vi "5.4-6.7.3-What Server.vi"() -> ()   [LabVIEW 2010]
doc: "Creates a named service and listens on the first available port. Whenever a client connects to the service, it responds with a message containing joystick data. The VI can be stopped using the STOP button."
uses:
  6-OCU Neurons/6.0-Super Heart Beat.ctl
  5.7-UDP/5.7 LabVIEW Errors.ctl
  5.0-Global.vi
panel:
  out "Super Heart Beat":T1
  in  "error in":errorcluster={"status"=TRUE, "code"=0, "source"=""}
  out "error out":errorcluster
  in  "stop":bool
  out "Probably a hello string":string
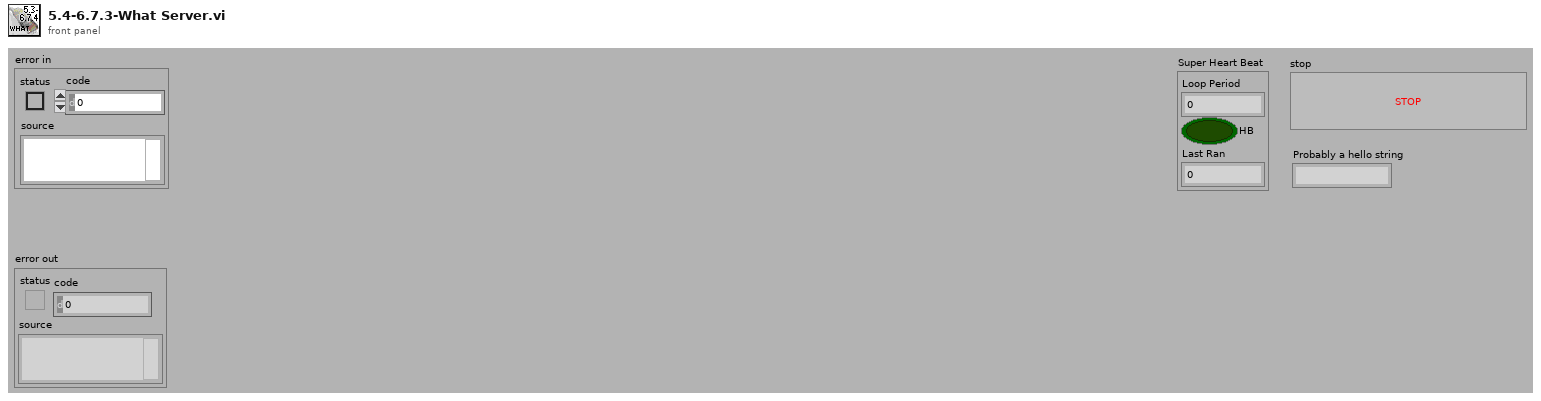
[diagram p1: front panel]
types:
  T1 = typedef "6.0-Super Heart Beat.ctl" = cluster{"Loop Period":u32, "HB":bool, "Last Ran":u32}
  T2 = typedef "6.3-What Reporting.ctl" = cluster{"LIDAR Data":T3}
  T3 = typedef "3.3.1-LIDAR Data Typedef.ctl" = cluster{"Angle array":dbl[], "Magnitude array ":dbl[]}
  T4 = typedef "5.7 LabVIEW Errors.ctl" = i32
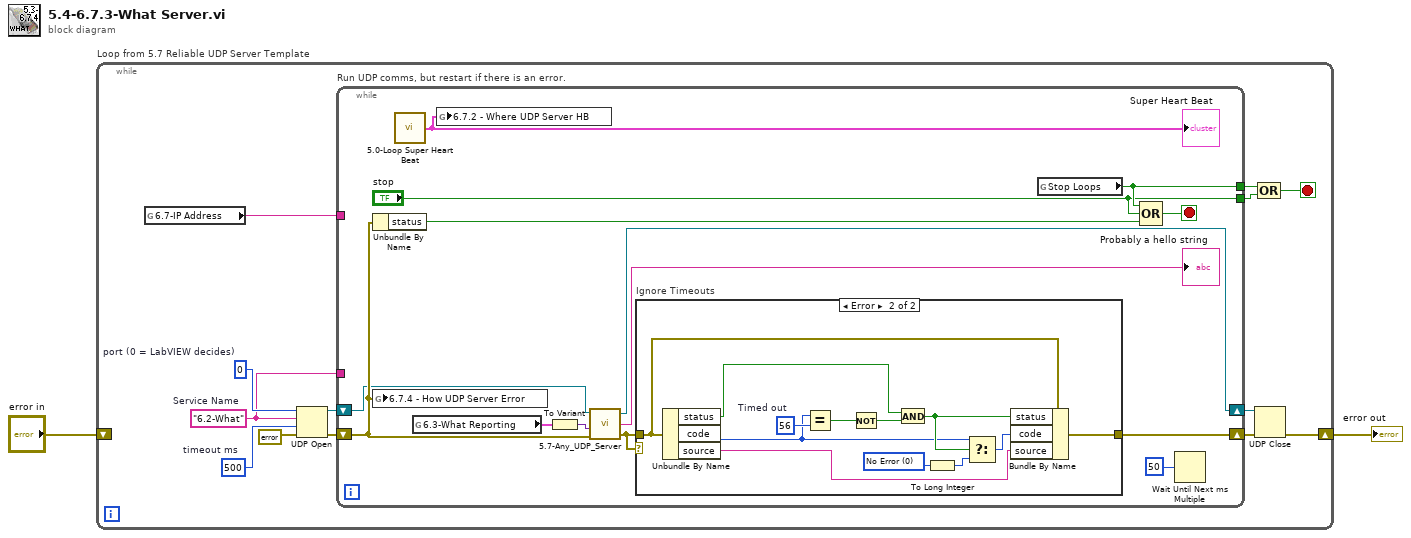
[diagram p0: block diagram]
diagram:
  n1 = while "Loop from 5.7 Reliable UDP Server Template" {
    shift-right: [w8] -> w1
    shift-left: "error in" -> [_]
    stop <- w13 stop-if-true
    w5 = 500  # timeout ms
    w7 = u16 0  # port (0 = LabVIEW decides)
    w6 = "6.2-What"  # Service Name
    n2 = global read "5.0-Global.vi" "6.7-IP Address"() -> (w4:string)
    n3 = UDP Open(8:errorcluster {"status"=FALSE, "code"=0, "source"=""} ("error in (no error)"), 9:w5, 10:w6, 11:w7) -> (port=w12:refnum<k16>, 0:w10:errorcluster)  [unwired: 1 in, 1 out]
    n4 = while "Run UDP comms, but restart if there is an error." {
      tunnel: w6 -> [_]
      tunnel: w4 -> [_]
      tunnel: [w27] -> w15
      tunnel: ["stop"] -> w14
      shift-right: [w20] -> w11
      shift-left: w12 -> [w21]
      shift-right: [w24] -> w9
      shift-left: w10 -> [w23]
      stop <- w29 stop-if-true
      n5 = Unbundle By Name(w23) -> ("status"=w25:bool)
      n6 = global write "5.0-Global.vi" "6.7.4 - How UDP Server Error"(w23) -> ()
      n7 = call "5.0-Loop Super Heart Beat.vi"() -> ("Super Heart Beat"=w16:T1)
      "Super Heart Beat" <- w16
      n8 = global read "5.0-Global.vi" "6.3-What Reporting"() -> (w17:T2)
      n9 = global write "5.0-Global.vi" "6.7.2 - Where UDP Server HB"(w16) -> ()
      n10 = To Variant(anything=w17) -> (Variant=w19:variant)
      n11 = call "5.7-Any_UDP_Server.vi"("error In"=w23, "Data in"=w19, "Connection ID"=w21) -> ("warning out"=w22:errorcluster, "data out"=→"Probably a hello string":string, "Connection ID out"=w20:refnum<k16>)  [unwired: 1 in]
      n12 = case "Ignore Timeouts" shown="Error" w22 {
        tunnel: w22 -> [w30 w42]
        tunnel: [w30 w41] -> w24
        frame No Error {
        }
        frame Error {
          w32 = T4 0 items=["No Error", "Argument Error", "Memory Full", "Out of Zone", "End of File", "File Already Open", "Generic File IO Error", "File Not Found", "File Permission Error", "Disk Full", "Duplicate Path", "Too Many Files Open", "Not Enabled", "Resource File Not Found", "Cannot Add Resource", "Resource Not Found", "Image Not Found", "Image Memory Error", "Pen Does Not Exist", "Config Bad Type", "Config Token Not Found", "Config Parse Error", "Config Memory Error", "Bad External Code Format", "Bad External Code Offset", "External Code Not Present", "Null Window", "Destroy Window Mixup", "Null Menu", "Print Aborted", "Bad Print Record", "Print Driver Error", "Windows Error During Print", "Memory Error During Print", "Print Dialog Error", "Generic Print Error", "Invalid Device Refnum", "Device Not Found", "Device Parameter Error", "Device Unit Error", "Can't Open Device", "Device Call Aborted", "Generic Error", "Cancelled By User", "Object ID Too Low", "Object ID Too High", "Object Not In Heap", "Unknown Heap", "Bad DefProc ID", "DefProc Not In Table", "Message Out Of Range", "Null Method", "Unknown Message", "Manager Call Not Supported", "Bad address", "Connection In progress", "Connection timed out", "Connection is already in progress", "Network attribute not supported", "Network error", "Address in use", "System out of memory", "Connection aborted", "Connection refused", "Connection is not connected", "Connection is already connected", "Connection closed", "Initialize error (interapplication manager)", "Bad occurrence", "Wait on unbound occurrence handler", "Occurrence queue overflow", "Bad path", "Semaphore not signaled", "Unrecognized type (interapplication manager)"] ("1st Error to Convert")
          w40 = 56  # Timed out
          n13 = Unbundle By Name(w42) -> ("status"=w37:bool, "code"=w35:i32, "source"=w33:string)
          n14 = Equal?(x=w35, y=w40) -> (x = y?=w39:bool)
          n15 = Not(x=w39) -> (.not. x?=w38:bool)
          n16 = And(x=w37, y=w38) -> (x .and. y?=w36:bool)
          n17 = To Long Integer(number=w32) -> (32bit integer=w31:T4)
          n18 = Select(t=w35, s=w36, f=w31) -> (s? t:f=w34:T4)
          n19 = Bundle By Name(cluster=w42, "status"=w36, "code"=w34, "source"=w33) -> (w41:errorcluster)
        }
      }
      n20 = global read "5.0-Global.vi" "Stop Loops"() -> (w27:bool)
      n21 = Compound Arithmetic op=OR(w27, "stop", w25) -> (w29:bool)
      n22 = Wait Until Next ms Multiple(millisecond multiple=u32 50) -> ()  [unwired: 1 out]
    }
    n23 = UDP Close(connection ID=w11, 8:w9) -> (error out=w8:errorcluster)  [unwired: 1 out]
    n24 = Compound Arithmetic op=OR(w15, w14) -> (w13:bool)
  }
  "error out" <- w1
